vi "Move.vi"(8 "error in (no error)":errorcluster, 10 "Amount (rev)":dbl, 11 "Dummy Motor in":refnum<class "Dummy Motor.lvclass">) -> (0 "error out":errorcluster, 3 "Dummy Motor out":refnum<class "Dummy Motor.lvclass">)   [LabVIEW 2015, in "Dummy Motor.lvclass"]
uses:
  Dummy Motor.lvclass
  Dummy Motor.lvclass/Dummy Motor.ctl
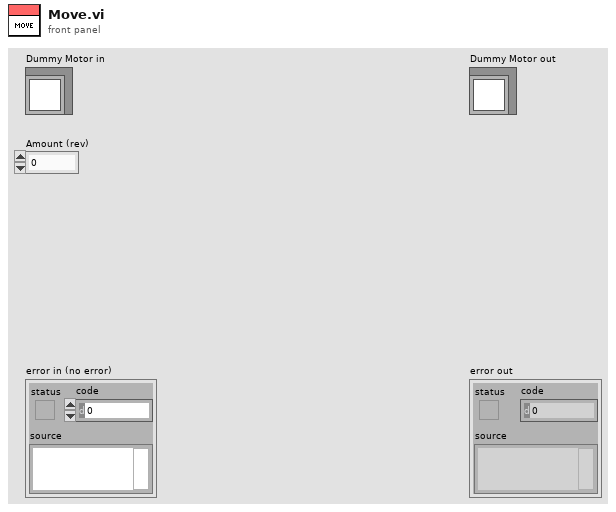
[diagram p1: front panel]
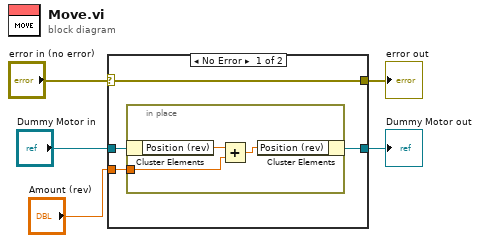
[diagram p0: block diagram]
diagram:
  n1 = case shown="No Error" "error in (no error)" {
    selector: "error in (no error)" -> [w9 w14]
    tunnel: [w9 w14] -> w3
    tunnel: [w7 w13] -> w2
    tunnel: "Dummy Motor in" -> [w8 w13]
    tunnel: "Amount (rev)" -> [w6 _]
    frame No Error {
      n2 = in-place {
        in-place-border: w6 -> [w11]
        n3 = in-place-cluster #1(w8) -> ("Position (rev)"=w12:dbl)
        n4 = Add(x=w12, y=w11) -> (x+y=w10:dbl)
        n5 = in-place-cluster #1("Position (rev)"=w10) -> (w7:refnum<class "Dummy Motor.lvclass">)
      }
    }
    frame Error {
    }
  }
  "error out" <- w3
  "Dummy Motor out" <- w2
